vi "主界面.vi"(0 "开始":bool, 5 "打开":bool, 9 "步骤":string[][](table)) -> (4 "T(cool)℃":string, 6 "P（eq)mv":string, 8 "多位阀的位置":string, 10 "R(Gas)mv":string, 15 "F(Flow)ml/min":string)   [LabVIEW 2016]
uses:
  <vilib>/Utility/miscctls.llb/LVRowAndColumnTypeDef.ctl
  <vilib>/Utility/file.llb/Write Delimited Spreadsheet (string).vi
  <vilib>/Utility/file.llb/Read Delimited Spreadsheet (string).vi
panel:
  out "报警":i32=1
  out "蠕动泵":i32=1
  out "电磁阀2":i32=1
  out "电磁阀1":i32=1
  out "气泵":i32=1
  out "时间":string
  out "d15N":string
  out "d15NA":string
  out "N2O":string
  out "d18O":string
  out "H2O  2":string
  out "温度摄氏度":string
  out "d15NB":string
  out "气压Torr":string
  out "超时us":string
  out "航向":string
  out "经度":string
  out "UTC日期":string
  out "速率":string
  out "纬度":string
  out "UTC时间":string
  out "定位信息":string
  in  "数据存储时间间隔（分钟）":dbl format="%#g"
  out "x*y":i32
  in  "数据数组":string[][](array[string])
  in  "停止":bool
  out "Delta2Min":string
  out "H2O":string
  out "12CO2":string
  out "12CO2(dry）":string
  out "13CO2":string
  out "13CO2（dry）":string
  out "Delta5Min":string
  out "Temperature":string
  out "Conductivity":string
  out "Salinity":string
  in  "设备配置&联机":bool
  out "跳转次数变量":i32=2
  out "当前步骤":i32
  in  "添加的数组 2":string[](array[string])
  out "编辑位置":T1
  in  "保存":bool
  in  "插入":bool
  in  "下移":bool
  in  "上移":bool
  in  "删除":bool
  out "数值 2":i32
  out "活动单元格:活动单元格":T1 caption="行和列"
  out "输出数组 2":string[][](array[string])
  in  "簇":T2
  in  "增加":bool
  in  "停止":bool
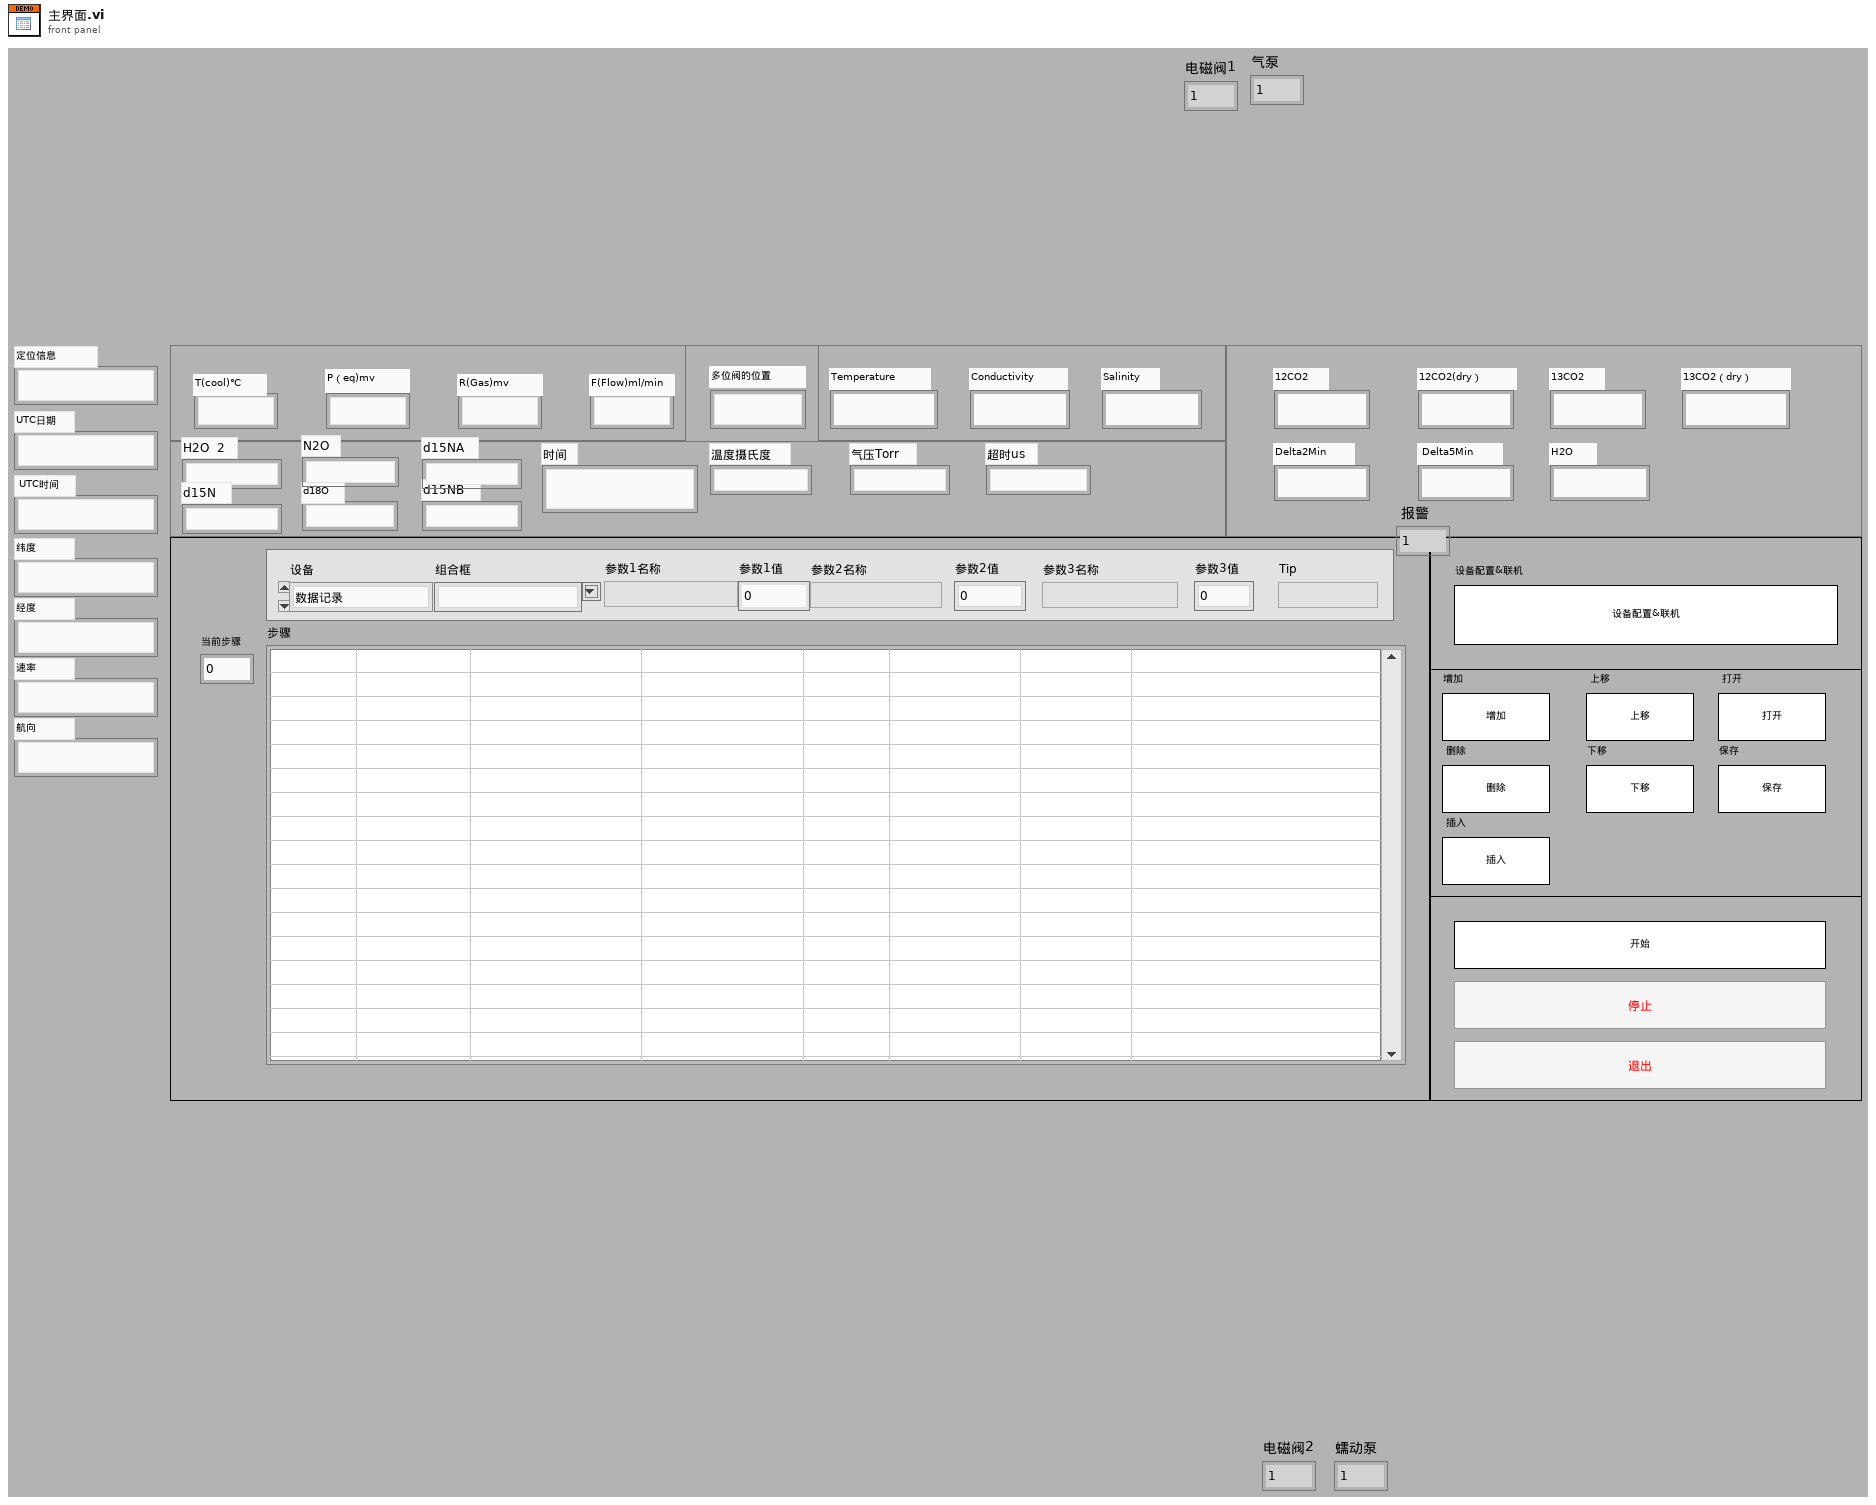
[diagram p1: front panel]
types:
  T1 = typedef "LVRowAndColumnTypeDef.ctl" = cluster{"Row":i32, "Column":i32}
  T2 = cluster{"设备":enum16{"数据记录", "Module", "VICI Valve", "其他"}, "组合框":string, "参数1名称":string, "参数1值":dbl, "参数2名称":string, "参数2值 ":dbl, "参数3名称 ":string, "参数3值  ":dbl, "Tip":string}
  T3 = typedef "LVPoint32TypeDef.ctl" = cluster{"Horizontal":i32, "Vertical":i32}
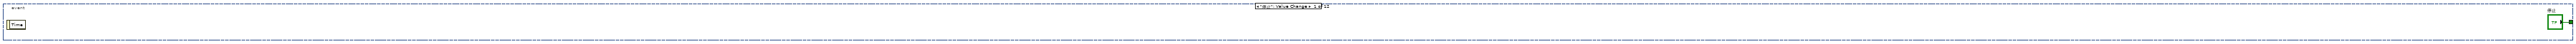
[diagram p2: hidden frame]
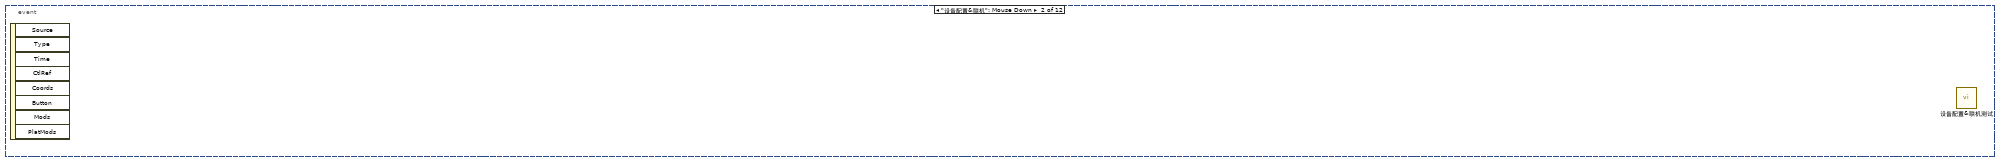
[diagram p3: hidden frame]
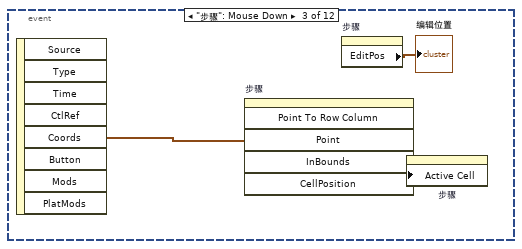
[diagram p4: hidden frame]
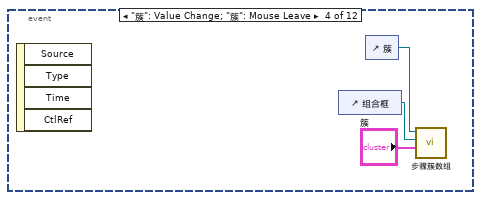
[diagram p5: hidden frame]
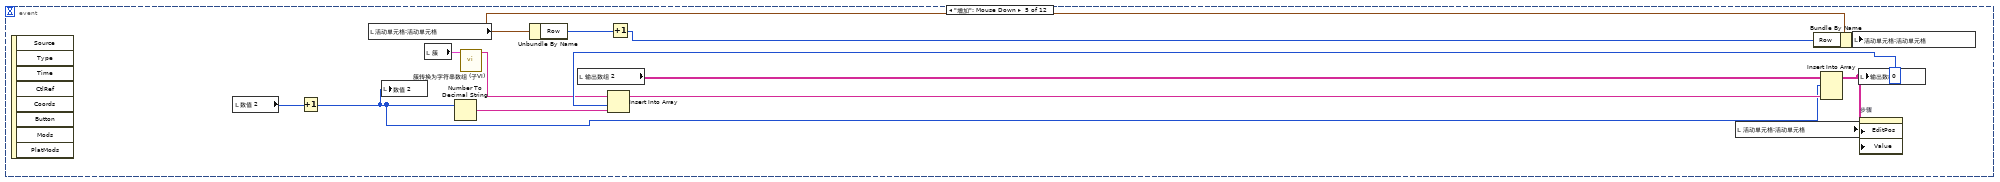
[diagram p6: hidden frame]
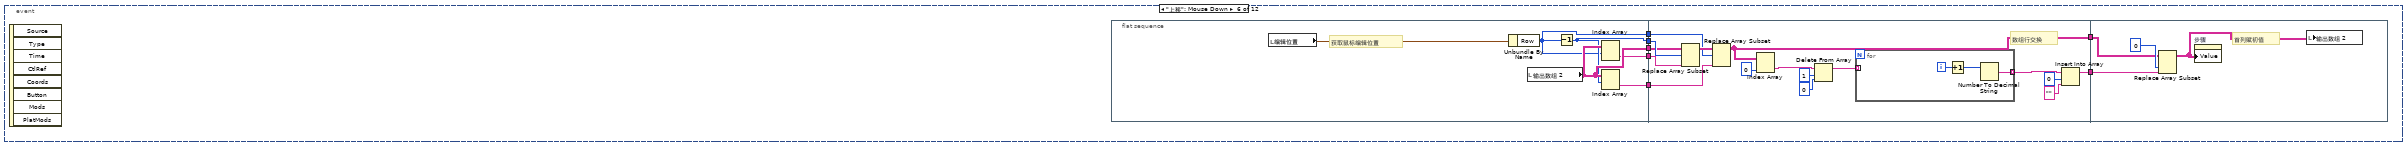
[diagram p7: hidden frame]
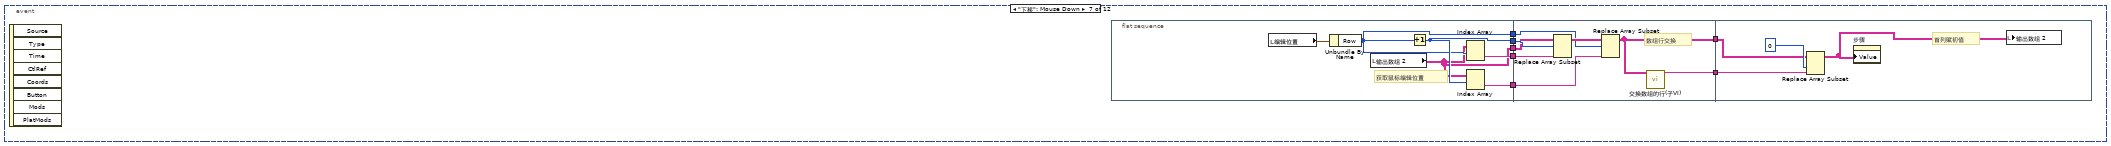
[diagram p8: hidden frame]
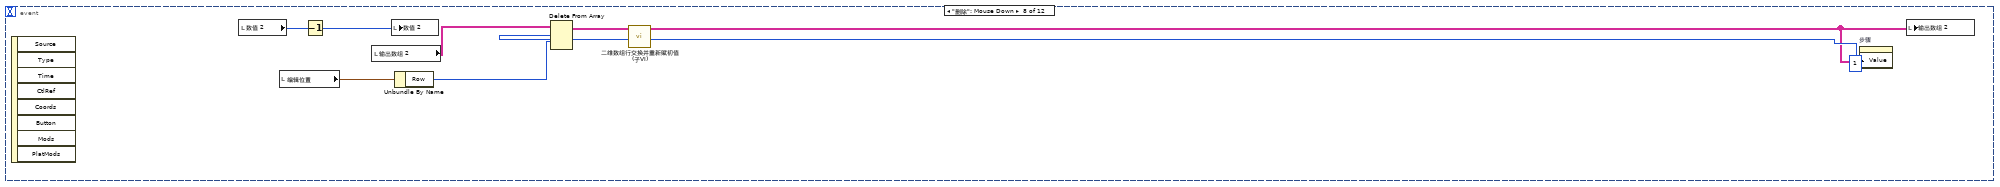
[diagram p9: hidden frame]
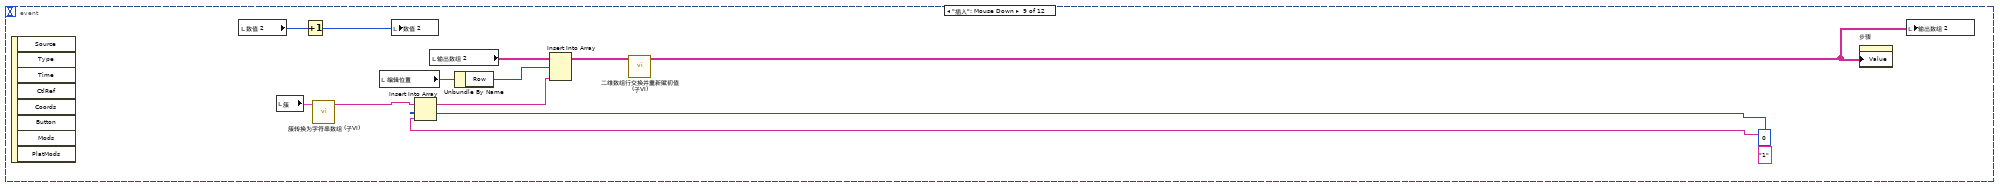
[diagram p10: hidden frame]
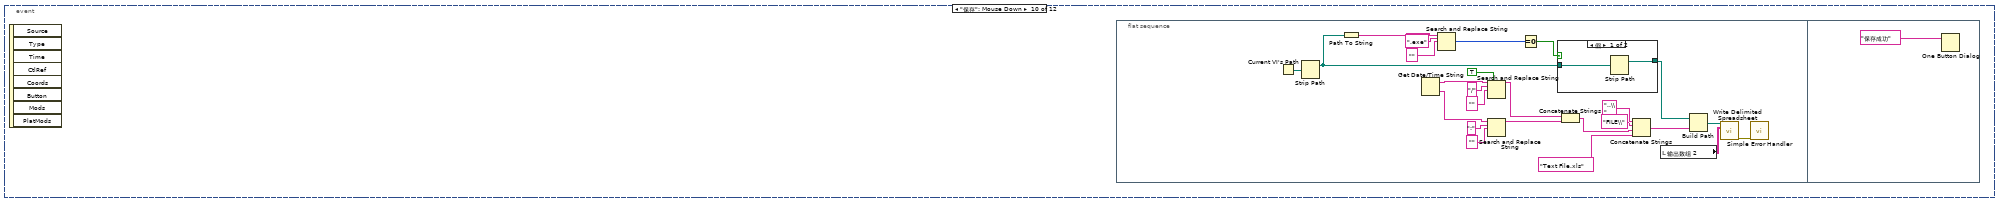
[diagram p11: hidden frame]
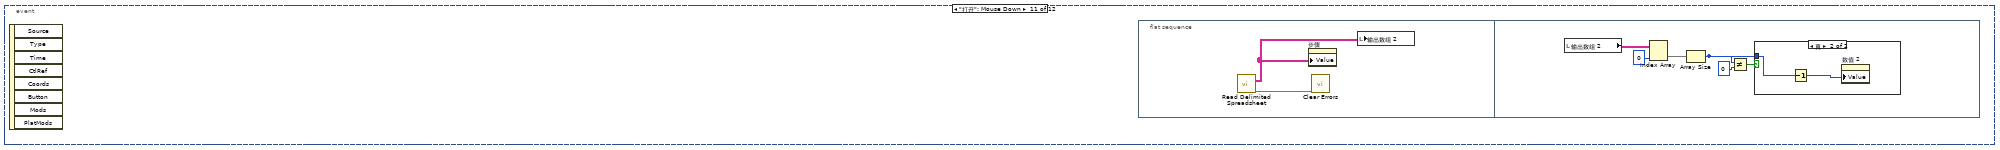
[diagram p13: hidden frame]
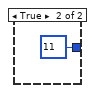
[diagram p15: hidden frame]
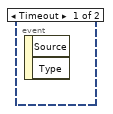
[diagram p17: hidden frame]
diagram:
  # "数组初始化"
  n1 = while {
    stop <- w40 stop-if-true
    w6 = FALSE ("停止")
    n2 = Wait (ms)(milliseconds to wait=u32 300 ("等待时间（毫秒）")) -> ()  [unwired: 1 out]
    n3 = event shown="[11] \"开始\": 鼠标按下" {
      selector: _ -> [_ _ _ _ _ _ _ _ _ _ _ _]
      dyn-events: _ -> [_ _ _ _ _ _ _ _ _ _ _ _]
      timeout: _ -> [_ _ _ _ _ _ _ _ _ _ _ _]
      tunnel: ["停止" _ _ _ _ _ _ _ _ _ _ _] -> w40
      event "停止": Value Change {
        n4 = event-data() -> ()  [unwired: 1 in, 1 out]
      }
      event "设备配置&联机": Mouse Down {
        n5 = event-data() -> ()  [unwired: 1 in, 8 out]
        n6 = call "设备配置&联机测试.vi"() -> ()  [unwired: 11 in, 1 out]
      }
      event "步骤": Mouse Down {
        n7 = event-data() -> ("Coords"=w44:T3)  [unwired: 1 in, 7 out]
        n8 = invoke on="步骤" class="Tbl (严格)" method="Point To Row Column"("Point"=w44) -> ("CellPosition"=w43:T1)  [unwired: 5 in, 5 out]
        n9 = property on="步骤" class="Tbl (严格)"() -> ("EditPos"=→"编辑位置":T1)  [unwired: 2 in, 2 out]
        n10 = property on="步骤" class="Tbl (严格)"("Active Cell"=w43) -> ()  [unwired: 2 in, 2 out]
      }
      event "簇": Value Change; "簇": Mouse Leave {
        n11 = event-data() -> ()  [unwired: 1 in, 4 out]
        n12 = control-ref of="组合框"() -> (w45:refnum<vi>)
        n13 = control-ref of="簇"() -> (w46:refnum<vi>)
        n14 = call "步骤簇数组.vi"("簇"="簇", "组合框"=w45, "簇 2"=w46) -> ()  [unwired: 9 in]
      }
      event "增加": Mouse Down {
        n15 = event-data() -> ()  [unwired: 1 in, 8 out]
        n16 = local read "数值 2"() -> (w53:i32)
        n17 = Increment(x=w53) -> (x+1=w52:i32)
        n18 = local read "活动单元格:活动单元格"() -> (w57:T1)
        n19 = local write "数值 2"(w52) -> ()
        n20 = local read "簇"() -> (w61:T2)
        n21 = Number To Decimal String(number=w52) -> (decimal integer string=w55:string)  [unwired: 1 in]
        n22 = call "簇转换为字符串数组 (子VI).vi"("簇"=w61) -> ("数组"=w48:string[])  [unwired: 10 in]
        n23 = Unbundle By Name(w57) -> ("Row"=w59:i32)
        n24 = local read "输出数组 2"() -> (w49:string[][])
        n25 = Insert Into Array(array=w48, index=0 ("索引"), new element=w55) -> (w54:string[])
        n26 = Increment(x=w59) -> (x+1=w56:i32)
        n27 = local read "活动单元格:活动单元格"() -> (w60:T1)
        n28 = Bundle By Name(cluster=w57, "Row"=w56) -> (w58:T1)
        n29 = Insert Into Array(array=w49, index (row)=w52, new element=w54) -> (w51:string[][])  [unwired: 1 in]
        n30 = local write "活动单元格:活动单元格"(w58) -> ()
        n31 = local write "输出数组 2"(w51) -> ()
        n32 = property on="步骤" class="Tbl (严格)"("EditPos"=w60, "Value"=w51) -> ()  [unwired: 2 in, 2 out]
      }
      event "上移": Mouse Down {
        n33 = event-data() -> ()  [unwired: 1 in, 8 out]
        n34 = flat-sequence {
          tunnel: [w73] -> w68
          tunnel: [w72] -> w67
          tunnel: [w71] -> w66
          tunnel: [w70] -> w65
          tunnel: [w69] -> w64
          tunnel: w68 -> [w77]
          tunnel: w67 -> [w90]
          tunnel: w66 -> [w89]
          tunnel: w65 -> [w87]
          tunnel: w64 -> [w86]
          tunnel: [w75] -> w63
          tunnel: [w76] -> w62
          tunnel: w63 -> [w96]
          tunnel: w62 -> [w95]
          frame #0 {
            # "获取鼠标编辑位置"
            n35 = local read "编辑位置"() -> (w74:T1)
            n36 = Unbundle By Name(w74) -> ("Row"=w69:i32)
            n37 = local read "输出数组 2"() -> (w73:string[][])
            n38 = Decrement(x=w69) -> (x-1=w71:i32)
            n39 = Index Array(array=w73, index (row)=w69) -> (element=w72:string[])  [unwired: 1 in]
            n40 = Index Array(array=w73, index (row)=w71) -> (element=w70:string[])  [unwired: 1 in]
          }
          frame #1 {
            # "数组行交换"
            n41 = Replace Array Subset(array=w77, new element=w90, index (row)=w89) -> (w88:string[][])  [unwired: 1 in]
            n42 = Replace Array Subset(array=w88, new element=w87, index (row)=w86) -> (w75:string[][])  [unwired: 1 in]
            n43 = Index Array(array=w75, index (col)=0 ("禁用的索引 (列)")) -> (element=w84:string[])  [unwired: 1 in]
            n44 = Delete From Array(array=w84, length=1 ("长度"), index=0 ("索引")) -> (array with subset deleted=w81:string[])  [unwired: 1 out]
            n45 = for {
              tunnel: w81 -> [_] mode=indexing
              tunnel: [w91] -> w80 mode=indexing
              i -> [w93]
              n46 = Increment(x=w93) -> (x+1=w92:i32)
              n47 = Number To Decimal String(number=w92) -> (decimal integer string=w91:string)  [unwired: 1 in]
            }
            n48 = Insert Into Array(array=w80, index=0 ("索引"), new element="" ("新元素/子数组")) -> (w76:string[])
          }
          frame #2 {
            # "首列赋初值"
            n49 = Replace Array Subset(array=w96, new element=w95, index (col)=0 ("禁用的索引 (列)")) -> (w94:string[][])  [unwired: 1 in]
            n50 = property on="步骤" class="Tbl (严格)"("Value"=w94) -> ()  [unwired: 2 in, 2 out]
            n51 = local write "输出数组 2"(w94) -> ()
          }
        }
      }
      event "下移": Mouse Down {
        n52 = event-data() -> ()  [unwired: 1 in, 8 out]
        n53 = flat-sequence {
          tunnel: [w105] -> w104
          tunnel: [w110] -> w103
          tunnel: [w109] -> w102
          tunnel: [w108] -> w101
          tunnel: [w107] -> w100
          tunnel: w104 -> [w113]
          tunnel: w103 -> [w118]
          tunnel: w102 -> [w117]
          tunnel: w101 -> [w115]
          tunnel: w100 -> [w114]
          tunnel: [w111] -> w99
          tunnel: [w112] -> w98
          tunnel: w99 -> [w121]
          tunnel: w98 -> [w120]
          frame #0 {
            # "获取鼠标编辑位置"
            n54 = local read "编辑位置"() -> (w106:T1)
            n55 = Unbundle By Name(w106) -> ("Row"=w107:i32)
            n56 = local read "输出数组 2"() -> (w105:string[][])
            n57 = Increment(x=w107) -> (x+1=w109:i32)
            n58 = Index Array(array=w105, index (row)=w107) -> (element=w110:string[])  [unwired: 1 in]
            n59 = Index Array(array=w105, index (row)=w109) -> (element=w108:string[])  [unwired: 1 in]
          }
          frame #1 {
            # "数组行交换"
            n60 = Replace Array Subset(array=w113, new element=w118, index (row)=w117) -> (w116:string[][])  [unwired: 1 in]
            n61 = Replace Array Subset(array=w116, new element=w115, index (row)=w114) -> (w111:string[][])  [unwired: 1 in]
            n62 = call "交换数组的行(子VI).vi"("输出数组输入"=w111) -> ("数组"=w112:string[])  [unwired: 10 in]
          }
          frame #2 {
            # "首列赋初值"
            n63 = Replace Array Subset(array=w121, new element=w120, index (col)=0 ("禁用的索引 (列)")) -> (w119:string[][])  [unwired: 1 in]
            n64 = property on="步骤" class="Tbl (严格)"("Value"=w119) -> ()  [unwired: 2 in, 2 out]
            n65 = local write "输出数组 2"(w119) -> ()
          }
        }
      }
      event "删除": Mouse Down {
        n66 = event-data() -> ()  [unwired: 1 in, 8 out]
        n67 = local read "数值 2"() -> (w126:i32)
        n68 = local read "编辑位置"() -> (w130:T1)
        n69 = Decrement(x=w126) -> (x-1=w125:i32)
        n70 = local read "输出数组 2"() -> (w129:string[][])
        n71 = local write "数值 2"(w125) -> ()
        n72 = Unbundle By Name(w130) -> ("Row"=w127:i32)
        n73 = Delete From Array(array=w129, length=1 ("长度"), index (row)=w127) -> (array with subset deleted=w124:string[][])  [unwired: 1 in, 1 out]
        n74 = call "二维数组行交换并重新赋初值 (子VI).vi"("输出数组 3"=w124) -> ("输出数组 2"=w123:string[][])  [unwired: 10 in]
        n75 = property on="步骤" class="Tbl (严格)"("Value"=w123) -> ()  [unwired: 2 in, 2 out]
        n76 = local write "输出数组 2"(w123) -> ()
      }
      event "插入": Mouse Down {
        n77 = event-data() -> ()  [unwired: 1 in, 8 out]
        n78 = local read "数值 2"() -> (w132:i32)
        n79 = local read "簇"() -> (w137:T2)
        n80 = Increment(x=w132) -> (x+1=w131:i32)
        n81 = call "簇转换为字符串数组 (子VI).vi"("簇"=w137) -> ("数组"=w136:string[])  [unwired: 10 in]
        n82 = local read "编辑位置"() -> (w142:T1)
        n83 = local write "数值 2"(w131) -> ()
        n84 = Insert Into Array(array=w136, index=0 ("索引"), new element="1" ("新元素/子数组")) -> (w133:string[])
        n85 = local read "输出数组 2"() -> (w141:string[][])
        n86 = Unbundle By Name(w142) -> ("Row"=w140:i32)
        n87 = Insert Into Array(array=w141, index (row)=w140, new element=w133) -> (w139:string[][])  [unwired: 1 in]
        n88 = call "二维数组行交换并重新赋初值 (子VI).vi"("输出数组 3"=w139) -> ("输出数组 2"=w138:string[][])  [unwired: 10 in]
        n89 = property on="步骤" class="Tbl (严格)"("Value"=w138) -> ()  [unwired: 2 in, 2 out]
        n90 = local write "输出数组 2"(w138) -> ()
      }
      event "保存": Mouse Down {
        n91 = event-data() -> ()  [unwired: 1 in, 8 out]
        n92 = flat-sequence {
          frame #0 {
            n93 = Current VI's Path() -> (path=w152:path)
            n94 = Strip Path(path=w152) -> (stripped path=w144:path)  [unwired: 1 out]
            n95 = Path To String(path=w144) -> (string=w149:string)
            n96 = Get Date/Time String() -> (date string=w160:string, time string=w163:string)  [unwired: 3 in]
            n97 = Search and Replace String(input string=w149, search string=".exe" ("搜索字符串"), replace string="" ("替换字符串(\"\")")) -> (number of replacements=w146:i32)  [unwired: 5 in, 3 out]
            n98 = Search and Replace String(input string=w163, search string=":" ("搜索字符串"), replace string="" ("替换字符串(\"\")")) -> (result string=w155:string)  [unwired: 5 in, 3 out]
            n99 = Search and Replace String(replace all?=TRUE ("替换全部？(F)"), input string=w160, search string="/" ("搜索字符串"), replace string="" ("替换字符串(\"\")")) -> (result string=w156:string)  [unwired: 4 in, 3 out]
            n100 = Equal To 0?(x=w146) -> (x = 0?=w145:bool)
            n101 = case shown="假" w145 {
              tunnel: w144 -> [w169 w170]
              tunnel: [w168 w170] -> w143
              frame False {
                n102 = Strip Path(path=w169) -> (stripped path=w168:path)  [unwired: 1 out]
              }
              frame True {
              }
            }
            n103 = Concatenate Strings(w156, w155) -> (w154:string)
            n104 = Concatenate Strings("..\\" ("字符串"), "FILE\\" ("替换字符串(\"\")"), w154, "Text File.xls" ("name or relative path")) -> (w165:string)
            n105 = local read "输出数组 2"() -> (w167:string[][])
            n106 = Build Path(base path=w143, name or relative path=w165) -> (appended path=w166:path)
            n107 = call-poly <vilib>:"Write Delimited Spreadsheet.vi"("file path (dialog if empty)"=w166, "2D data"=w167) -> ("error out"=w153:errorcluster)  [unwired: 12 in, 1 out]
            n108 = call <vilib>:"Simple Error Handler.vi"("error in (no error)"=w153) -> ()  [unwired: 4 in, 5 out]
          }
          frame #1 {
            n109 = One Button Dialog(message="保存成功" ("消息")) -> ()  [unwired: 1 in, 1 out]
          }
        }
      }
      event "打开": Mouse Down {
        n110 = event-data() -> ()  [unwired: 1 in, 8 out]
        n111 = flat-sequence {
          frame #0 {
            n112 = call-poly <vilib>:"Read Delimited Spreadsheet.vi"() -> ("all rows"=w173:string[][], "error out"=w172:errorcluster)  [unwired: 10 in, 4 out]
            n113 = property on="步骤" class="Tbl (严格)"("Value"=w173) -> ()  [unwired: 2 in, 2 out]
            n114 = call <vilib>:"Clear Errors.vi"("error in (no error)"=w172) -> ()  [unwired: 5 in, 2 out]
            n115 = local write "输出数组 2"(w173) -> ()
          }
          frame #1 {
            n116 = local read "输出数组 2"() -> (w177:string[][])
            n117 = Index Array(array=w177, index (col)=0 ("禁用的索引 (列)")) -> (element=w175:string[])  [unwired: 1 in]
            n118 = Array Size(array=w175) -> (size(s)=w174:i32)
            n119 = Not Equal?(x=w174, y=u32 0) -> (x != y?=w178:bool)
            n120 = case shown="真" w178 {
              tunnel: w174 -> [_ w181]
              frame False {
              }
              frame True {
                n121 = Decrement(x=w181) -> (x-1=w180:i32)
                n122 = property on="数值 2" class="DigNum (严格)"("Value"=w180) -> ()  [unwired: 2 in, 2 out]
              }
            }
          }
        }
      }
      event "开始": Mouse Down {
        w182 = 0 ("气泵")
        w184 = ""
        n123 = event-data() -> ()  [unwired: 1 in, 8 out]
        n124 = while {
          stop <- w215 stop-if-true
          # "数据显示"
          # "读取流量传感器"
          n125 = call "读取流量传感器(子VI).vi"() -> ("结果"=w216:bool, "R(Gas)mv"=w221:string, "F(Flow)ml/min"=w220:string, "P（eq)mv"=w222:string, "T(cool)℃"=w223:string)  [unwired: 7 in]
          n126 = local write "P（eq)mv"(w222) -> ()
          n127 = local write "R(Gas)mv"(w221) -> ()
          n128 = local write "F(Flow)ml/min"(w220) -> ()
          n129 = local write "T(cool)℃"(w223) -> ()
          n130 = disable-structure shown="禁用" {
            frame Disabled {
              n131 = call "N2O同位素分析仪串口通讯.vi"("VISA resource name"=refnum<visa-resource-name> "COM8") -> ("温度摄氏度"=→"温度摄氏度":string, "d15NB"=→"d15NB":string, "时间"=→"时间":string, "N2O"=→"N2O":string, "d15N"=→"d15N":string, "d18O"=→"d18O":string, "超时us"=→"超时us":string, "气压Torr"=→"气压Torr":string, "H2O"=→"H2O  2":string, "d15NA"=→"d15NA":string)  [unwired: 5 in]
            }
            frame Enabled {
            }
          }
          n132 = call "SBE45通讯参数 (子VI).vi"() -> ("错误输出"=w214:errorcluster, "Salinity"=w238:string, "Conductivity"=w239:string, "Temperature"=w240:string)  [unwired: 8 in]
          "Temperature" <- w240
          "Conductivity" <- w239
          "Salinity" <- w238
          n133 = call "G2131-i通讯参数 (子VI).vi"() -> ("12CO2(dry）"=w235:string, "Delta2Min"=w231:string, "12CO2"=w236:string, "Delta5Min"=w230:string, "H2O"=w232:string, "13CO2"=w234:string, "13CO2（dry）"=w233:string)  [unwired: 5 in]
          "Delta2Min" <- w231
          "H2O" <- w232
          "12CO2" <- w236
          "12CO2(dry）" <- w235
          "13CO2" <- w234
          "13CO2（dry）" <- w233
          "Delta5Min" <- w230
          n134 = local read "多位阀的位置"() -> (w241:string)
          n135 = Get Date/Time String(want seconds? (F)=TRUE ("需要秒？(F)")) -> (date string=w227:string, time string=w229:string)  [unwired: 2 in]
          n136 = Concatenate Strings(w227, " " ("字符串"), w229) -> (w205:string)
          n137 = call "GPS-1仪器串口通讯.vi"("VISA resource name"=refnum<visa-resource-name> "COM5", "baud rate (9600)"=u32 9600) -> ("速率"=w211:string, "经度"=w210:string, "定位信息"=w206:string, "UTC日期"=w207:string, "航向"=w212:string, "UTC时间"=w208:string, "纬度"=w209:string)  [unwired: 10 in, 1 out]
          "定位信息" <- w206
          "UTC时间" <- w208
          "纬度" <- w209
          "速率" <- w211
          "UTC日期" <- w207
          "经度" <- w210
          "航向" <- w212
          n138 = Compound Arithmetic op=OR ("复合运算")(w214, w216, "停止") -> (w215:bool)
          n139 = Build Array(w205, w206, w207, w208, w209, w210, w211, w212, w223, w222, w221, w220, w241, w240, w239, w238, w236, w235, w234, w233, w232, w231, w230) -> (w237:string[])
          n140 = Insert Into Array(array="数据数组", index (row)=2 ("索引 (行)"), new element=w237) -> (w213:string[][])  [unwired: 1 in]
          n141 = local write "数据数组"(w213) -> ()
          n142 = case shown="假" "停止" {
            tunnel: [w242 11 ("x*y")] -> w217
            frame False {
              n143 = local read "x*y"() -> (w242:i32)
            }
            frame True {
            }
          }
          n144 = Wait (ms)(milliseconds to wait=w217) -> ()  [unwired: 1 out]
        }
        n145 = local read "输出数组 2"() -> (w203:string[][])
        n146 = local write "F(Flow)ml/min"(w184) -> ()
        n147 = local write "P（eq)mv"(w184) -> ()
        n148 = local write "T(cool)℃"(w184) -> ()
        n149 = local write "R(Gas)mv"(w184) -> ()
        n150 = call "提示用户输入"() -> ("数据存储时间间隔（分钟）"=w183:dbl)  [unwired: 17 in, 2 out]
        n151 = call "二维数组行交换并重新赋初值 (子VI).vi"("输出数组 3"=w203) -> ("输出数组 2"=w202:string[][])  [unwired: 10 in]
        n152 = Delete From Array(array=w202, index (row)=0 ("索引 (行)")) -> (array with subset deleted=w190:string[][])  [unwired: 2 in, 1 out]
        n153 = local write "数据存储时间间隔（分钟）"(w183) -> ()
        n154 = Index Array(array=w190, index (col)=2 ("禁用的索引 (列)")) -> (element=w199:string[])  [unwired: 1 in]
        n155 = Index Array(array=w190, index (col)=4 ("禁用的索引 (列)")) -> (element=w200:string[])  [unwired: 1 in]
        n156 = Index Array(array=w190, index (col)=6 ("禁用的索引 (列)")) -> (element=w188:string[])  [unwired: 1 in]
        n157 = local write "电磁阀2"(w182) -> ()
        n158 = local write "电磁阀1"(w182) -> ()
        n159 = local write "报警"(w182) -> ()
        n160 = local write "蠕动泵"(w182) -> ()
        n161 = local write "气泵"(w182) -> ()
        n162 = Build Array(w199, w200, w188) -> (w192:string[][])
        n163 = Obtain Queue(name (unnamed)="步骤执行顺序数组" ("名称（未命名）"), element data type="添加的数组 2") -> (queue out=w193:refnum<queue>, error out=w186:errorcluster)  [unwired: 3 in, 1 out]
        n164 = while {
          tunnel: w192 -> [w325]
          tunnel: [w323] -> w194
          tunnel: w193 -> [w318]
          tunnel: w186 -> [w296]
          tunnel: [w287] -> w185
          stop <- w255 stop-if-true
          n165 = event shown="[1] \"当前步骤\": 值改变" {
            selector: _ -> [_ _]
            dyn-events: _ -> [_ _]
            timeout: _ -> [_ _]
            event Timeout {
              n166 = event-data() -> ()  [unwired: 1 in, 2 out]
            }
            event "当前步骤": Value Change {
              n167 = event-data() -> ()  [unwired: 1 in, 6 out]
              n168 = control-ref of="步骤"() -> (w328:refnum<vi>)
              n169 = property on="当前步骤" class="DigNum (严格)"() -> ("Value"=w327:i32)  [unwired: 2 in, 2 out]
              n170 = Bundle By Name(cluster=T1 {"Row"=0, "Column"=-2} ("活动单元格:活动单元格"), "Row"=w327) -> (w331:T1)
              n171 = property class="Tbl (严格)"(reference=w328, "Cell BG Color"=u32 16448250, "Active Cell"=w331, "Cell BG Color"=u32 3381759) -> ()  [unwired: 1 in, 2 out]
            }
          }
          n172 = Get Queue Status(queue=w318) -> ()  [unwired: 2 in, 8 out]
          n173 = Wait (ms)(milliseconds to wait=u32 3000 ("等待时间（毫秒）")) -> ()  [unwired: 1 out]
          n174 = local read "当前步骤"() -> (w319:i32)
          n175 = Index Array(array=w325, index (col)=w319) -> (element=w317:string[])  [unwired: 1 in]
          n176 = Increment(x=w319) -> (x+1=w258:i32)
          n177 = Empty Array?(array=w317) -> (empty?=w259:bool)
          n178 = Enqueue Element(queue=w318, element=w317, error in (no error)=w296) -> (queue out=w326:refnum<queue>, error out=w297:errorcluster)  [unwired: 1 in, 1 out]
          n179 = property on="当前步骤" class="DigNum (严格)"("Val(Sgnl)"=w258) -> ()  [unwired: 2 in, 2 out]
          n180 = Dequeue Element(queue=w326, error in (no error)=w297) -> (queue out=w323:refnum<queue>, element=w265:string[], error out=w287:errorcluster)  [unwired: 1 in, 1 out]
          n181 = Index Array(array=w265, index=0 ("索引")) -> (element=w262:string)
          n182 = Equal?(x=w262, y="Control Devices") -> (x = y?=w274:bool)
          n183 = Equal?(x=w262, y="Read Alarm ") -> (x = y?=w270:bool)
          n184 = Equal?(x=w262, y="Set Valve Position") -> (x = y?=w303:bool)
          n185 = Equal?(x=w262, y="Read All sensor Values") -> (x = y?=w304:bool)
          n186 = Equal?(x=w262, y="暂停") -> (x = y?=w261:bool)
          n187 = Equal?(x=w262, y="恢复") -> (x = y?=w260:bool)
          n188 = Equal?(x=w262, y="等待") -> (x = y?=w299:bool)
          n189 = Equal?(x=w262, y="开始") -> (x = y?=w266:bool)
          n190 = Equal?(x=w262, y="跳转事件") -> (x = y?=w320:bool)
          n191 = Equal?(x=w262, y="气泵1、2") -> (x = y?=w316:bool)
          n192 = Equal?(x=w262, y="电磁阀1") -> (x = y?=w315:bool)
          n193 = Equal?(x=w262, y="电磁阀2") -> (x = y?=w312:bool)
          n194 = Equal?(x=w262, y="蠕动泵") -> (x = y?=w311:bool)
          n195 = Equal?(x=w262, y="报警器开") -> (x = y?=w308:bool)
          n196 = Equal?(x=w262, y="报警器关") -> (x = y?=w307:bool)
          n197 = Equal?(x=w262, y="单次记录") -> (x = y?=w268:bool)
          n198 = Or(x=w274, y=w270) -> (x .or. y?=w273:bool)
          n199 = case shown="真" w311 {
            tunnel: w265 -> [_ w478]
            tunnel: [_ w476] -> w293
            frame False {
            }
            frame True {
              # "蠕动泵"
              n200 = Index Array(array=w478, index=1 ("索引")) -> (element=w480:string)
              n201 = Equal?(x=w480, y="1") -> (x = y?=w477:bool)
              n202 = case shown="真" w477 {
                tunnel: [_ w497] -> w476
                tunnel: [0 ("电磁阀1") 10 ("电磁阀1")] -> w475
                frame False {
                  n203 = disable-structure shown="禁用" {
                    disable-tunnel: [w483 _] -> _
                    frame Disabled {
                      n204 = call "Module仪器串口通讯.vi"("输入指令"="$3DO00\r", "baud rate"=u32 300 ("baud rate (9600)"), "VISA resource name"=refnum<visa-resource-name> "COM3") -> ("错误输出"=w483:errorcluster)  [unwired: 2 out]
                    }
                    frame Enabled {
                    }
                  }
                }
                frame True {
                  n205 = control-ref of="电磁阀2"() -> (w493:refnum<vi>)
                  n206 = control-ref of="电磁阀1"() -> (w495:refnum<vi>)
                  n207 = control-ref of="报警"() -> (w494:refnum<vi>)
                  n208 = control-ref of="气泵"() -> (w492:refnum<vi>)
                  n209 = call "数值连接 (子VI).vi"("DigNum引用句柄 4"=w495, "x"=10, "DigNum引用句柄 3"=w494, "DigNum引用句柄输入"=w493, "Digital输入"=w492) -> ("数据字符串"=w490:string)  [unwired: 6 in]
                  n210 = Replace Substring(2:2 ("长度（子字符串长度）"), 3:4 ("偏移量(0)"), 4:w490, 5:"$3DO10\r" ("输入指令")) -> (1:w489:string)  [unwired: 1 out]
                  n211 = call "Module仪器串口通讯.vi"("输入指令"=w489, "baud rate"=u32 300 ("baud rate (9600)"), "VISA resource name"=refnum<visa-resource-name> "COM3") -> ("错误输出"=w497:errorcluster)  [unwired: 2 out]
                }
              }
              "蠕动泵" <- w475
            }
          }
          n212 = case shown="真" w261 {
            frame False {
            }
            frame True {
              n213 = local read "当前步骤"() -> (w336:i32)
              n214 = Increment(x=w336) -> (x+1=w335:i32)
              n215 = property on="当前步骤" class="DigNum (严格)"("Val(Sgnl)"=w335) -> ()  [unwired: 2 in, 2 out]
            }
          }
          n216 = case shown="真" w260 {
            frame False {
            }
            frame True {
              n217 = local read "当前步骤"() -> (w334:i32)
              n218 = Increment(x=w334) -> (x+1=w333:i32)
              n219 = property on="当前步骤" class="DigNum (严格)"("Val(Sgnl)"=w333) -> ()  [unwired: 2 in, 2 out]
            }
          }
          n220 = case shown="真" w273 {
            frame False {
            }
            frame True {
              n221 = local read "当前步骤"() -> (w387:i32)
              n222 = Increment(x=w387) -> (x+1=w386:i32)
              n223 = property on="当前步骤" class="DigNum (严格)"("Val(Sgnl)"=w386) -> ()  [unwired: 2 in, 2 out]
            }
          }
          n224 = case shown="真" w299 {
            tunnel: w265 -> [_ w392]
            frame False {
            }
            frame True {
              n225 = Index Array(array=w392, index=1 ("索引")) -> (element=w391:string)
              n226 = Decimal String To Number(string=w391) -> (number=w390:i32)  [unwired: 2 in, 1 out]
              n227 = Multiply(x=w390, y=60000) -> (x*y=w388:i32)
              n228 = Wait (ms)(milliseconds to wait=w388) -> ()  [unwired: 1 out]
            }
          }
          n229 = case shown="真" w316 {
            tunnel: w265 -> [_ w554]
            tunnel: [_ w552] -> w298
            frame False {
            }
            frame True {
              # "气泵"
              n230 = Index Array(array=w554, index=1 ("索引")) -> (element=w556:string)
              n231 = Equal?(x=w556, y="1") -> (x = y?=w553:bool)
              n232 = case shown="真" w553 {
                tunnel: [_ w574] -> w552
                tunnel: [0 1] -> w551
                frame False {
                  n233 = disable-structure shown="禁用" {
                    disable-tunnel: [w559 _] -> _
                    frame Disabled {
                      n234 = call "Module仪器串口通讯.vi"("输入指令"="$3DO00\r", "baud rate"=u32 300 ("baud rate (9600)"), "VISA resource name"=refnum<visa-resource-name> "COM3") -> ("错误输出"=w559:errorcluster)  [unwired: 2 out]
                    }
                    frame Enabled {
                    }
                  }
                }
                frame True {
                  n235 = control-ref of="电磁阀2"() -> (w568:refnum<vi>)
                  n236 = control-ref of="电磁阀1"() -> (w569:refnum<vi>)
                  n237 = control-ref of="蠕动泵"() -> (w570:refnum<vi>)
                  n238 = control-ref of="报警"() -> (w571:refnum<vi>)
                  n239 = call "数值连接 (子VI).vi"("DigNum引用句柄 4"=w571, "x"=1, "DigNum引用句柄 3"=w570, "DigNum引用句柄输入"=w569, "Digital输入"=w568) -> ("数据字符串"=w567:string)  [unwired: 6 in]
                  n240 = Replace Substring(2:2 ("长度（子字符串长度）"), 3:4 ("偏移量(0)"), 4:w567, 5:"$3DO01\r" ("输入指令")) -> (1:w564:string)  [unwired: 1 out]
                  n241 = call "Module仪器串口通讯.vi"("输入指令"=w564, "baud rate"=u32 300 ("baud rate (9600)"), "VISA resource name"=refnum<visa-resource-name> "COM3") -> ("错误输出"=w574:errorcluster)  [unwired: 2 out]
                }
              }
              "气泵" <- w551
            }
          }
          n242 = case shown="真" w315 {
            tunnel: w265 -> [_ w529]
            tunnel: [_ w527] -> w291
            frame False {
            }
            frame True {
              # "电磁阀1"
              n243 = Index Array(array=w529, index=1 ("索引")) -> (element=w531:string)
              n244 = Equal?(x=w531, y="1") -> (x = y?=w528:bool)
              n245 = case shown="真" w528 {
                tunnel: [_ w547] -> w527
                tunnel: [0 ("电磁阀1") 4 ("电磁阀1")] -> w526
                frame False {
                  n246 = disable-structure shown="禁用" {
                    frame Disabled {
                      n247 = call "Module仪器串口通讯.vi"("输入指令"="$3DO00\r", "baud rate"=u32 300 ("baud rate (9600)"), "VISA resource name"=refnum<visa-resource-name> "COM3") -> ()  [unwired: 3 out]
                    }
                    frame Enabled {
                    }
                  }
                }
                frame True {
                  n248 = control-ref of="电磁阀2"() -> (w540:refnum<vi>)
                  n249 = control-ref of="蠕动泵"() -> (w541:refnum<vi>)
                  n250 = control-ref of="报警"() -> (w539:refnum<vi>)
                  n251 = control-ref of="气泵"() -> (w542:refnum<vi>)
                  n252 = call "数值连接 (子VI).vi"("DigNum引用句柄 4"=w539, "x"=4, "DigNum引用句柄 3"=w540, "DigNum引用句柄输入"=w541, "Digital输入"=w542) -> ("数据字符串"=w545:string)  [unwired: 6 in]
                  n253 = Replace Substring(2:2 ("长度（子字符串长度）"), 3:4 ("偏移量(0)"), 4:w545, 5:"$3DO04\r" ("输入指令")) -> (1:w538:string)  [unwired: 1 out]
                  n254 = call "Module仪器串口通讯.vi"("输入指令"=w538, "baud rate"=u32 300 ("baud rate (9600)"), "VISA resource name"=refnum<visa-resource-name> "COM3") -> ("错误输出"=w547:errorcluster)  [unwired: 2 out]
                }
              }
              "电磁阀1" <- w526
            }
          }
          n255 = case shown="真" w320 {
            tunnel: w265 -> [_ w577]
            frame False {
            }
            frame True {
              # "跳转次数"
              n256 = Index Array(array=w577, index=2 ("索引")) -> (element=w582:string)
              n257 = local read "跳转次数变量"() -> (w581:i32)
              n258 = Decimal String To Number(string=w582) -> (number=w578:i32)  [unwired: 2 in, 1 out]
              n259 = Increment(x=w581) -> (x+1=w580:i32)
              n260 = local write "跳转次数变量"(w580) -> ()
              n261 = Greater Or Equal?(x=w580, y=w578) -> (x >= y?=w579:bool)
              n262 = case shown="真" w579 {
                tunnel: w577 -> [w584 _]
                frame False {
                  # "跳转"
                  n263 = Index Array(array=w584, index=1 ("索引")) -> (element=w586:string)
                  n264 = Decimal String To Number(string=w586) -> (number=w587:i32)  [unwired: 2 in, 1 out]
                  n265 = property on="当前步骤" class="DigNum (严格)"("Val(Sgnl)"=w587) -> ()  [unwired: 2 in, 2 out]
                }
                frame True {
                  n266 = local read "当前步骤"() -> (w589:i32)
                  n267 = Increment(x=w589) -> (x+1=w588:i32)
                  n268 = property on="当前步骤" class="DigNum (严格)"("Val(Sgnl)"=w588) -> ()  [unwired: 2 in, 2 out]
                }
              }
            }
          }
          n269 = case shown="真" w312 {
            tunnel: w265 -> [_ w504]
            tunnel: [_ w502] -> w292
            frame False {
            }
            frame True {
              # "电磁阀2"
              n270 = Index Array(array=w504, index=1 ("索引")) -> (element=w506:string)
              n271 = Equal?(x=w506, y="1") -> (x = y?=w503:bool)
              n272 = case shown="真" w503 {
                tunnel: [_ w523] -> w502
                tunnel: [0 ("电磁阀1") 8 ("电磁阀1")] -> w501
                frame False {
                  n273 = disable-structure shown="禁用" {
                    frame Disabled {
                      n274 = call "Module仪器串口通讯.vi"("输入指令"="$3DO00\r", "baud rate"=u32 300 ("baud rate (9600)"), "VISA resource name"=refnum<visa-resource-name> "COM3") -> ()  [unwired: 3 out]
                    }
                    frame Enabled {
                    }
                  }
                }
                frame True {
                  n275 = control-ref of="报警"() -> (w512:refnum<vi>)
                  n276 = control-ref of="电磁阀1"() -> (w514:refnum<vi>)
                  n277 = control-ref of="蠕动泵"() -> (w513:refnum<vi>)
                  n278 = control-ref of="气泵"() -> (w515:refnum<vi>)
                  n279 = call "数值连接 (子VI).vi"("DigNum引用句柄 4"=w512, "x"=8, "DigNum引用句柄 3"=w513, "DigNum引用句柄输入"=w514, "Digital输入"=w515) -> ("数据字符串"=w516:string)  [unwired: 6 in]
                  n280 = Replace Substring(2:2 ("长度（子字符串长度）"), 3:4 ("偏移量(0)"), 4:w516, 5:"$3DO08\r" ("输入指令")) -> (1:w521:string)  [unwired: 1 out]
                  n281 = call "Module仪器串口通讯.vi"("输入指令"=w521, "baud rate"=u32 300 ("baud rate (9600)"), "VISA resource name"=refnum<visa-resource-name> "COM3") -> ("错误输出"=w523:errorcluster)  [unwired: 2 out]
                }
              }
              "电磁阀2" <- w501
            }
          }
          n282 = case shown="真" w308 {
            tunnel: w265 -> [_ w452]
            tunnel: [_ w450] -> w294
            frame False {
            }
            frame True {
              # "报警器"
              n283 = Index Array(array=w452, index=1 ("索引")) -> (element=w454:string)
              n284 = Equal?(x=w454, y="1") -> (x = y?=w451:bool)
              n285 = case shown="真" w451 {
                tunnel: [_ w471] -> w450
                tunnel: [0 ("电磁阀1") 40 ("电磁阀1")] -> w449
                frame False {
                  n286 = disable-structure shown="禁用" {
                    disable-tunnel: [w457 _] -> _
                    frame Disabled {
                      n287 = call "Module仪器串口通讯.vi"("输入指令"="$3DO00\r", "baud rate"=u32 300 ("baud rate (9600)"), "VISA resource name"=refnum<visa-resource-name> "COM3") -> ("错误输出"=w457:errorcluster)  [unwired: 2 out]
                    }
                    frame Enabled {
                    }
                  }
                }
                frame True {
                  n288 = control-ref of="电磁阀2"() -> (w468:refnum<vi>)
                  n289 = control-ref of="蠕动泵"() -> (w467:refnum<vi>)
                  n290 = control-ref of="电磁阀1"() -> (w466:refnum<vi>)
                  n291 = control-ref of="气泵"() -> (w469:refnum<vi>)
                  n292 = call "数值连接 (子VI).vi"("DigNum引用句柄 4"=w466, "x"=4, "DigNum引用句柄 3"=w467, "DigNum引用句柄输入"=w468, "Digital输入"=w469) -> ("数据字符串"=w463:string)  [unwired: 6 in]
                  n293 = Replace Substring(2:2 ("长度（子字符串长度）"), 3:4 ("偏移量(0)"), 4:w463, 5:"$3DO40\r" ("输入指令")) -> (1:w465:string)  [unwired: 1 out]
                  n294 = call "Module仪器串口通讯.vi"("输入指令"=w465, "baud rate"=u32 300 ("baud rate (9600)"), "VISA resource name"=refnum<visa-resource-name> "COM3") -> ("错误输出"=w471:errorcluster)  [unwired: 2 out]
                }
              }
              "报警" <- w449
            }
          }
          n295 = case shown="真" w307 {
            tunnel: w265 -> [_ w437]
            tunnel: [_ w435] -> w295
            frame False {
            }
            frame True {
              n296 = Index Array(array=w437, index=1 ("索引")) -> (element=w439:string)
              n297 = Equal?(x=w439, y="1") -> (x = y?=w436:bool)
              n298 = case shown="真" w436 {
                tunnel: [_ w445] -> w435
                frame False {
                  n299 = disable-structure shown="禁用" {
                    disable-tunnel: [w441 _] -> _
                    frame Disabled {
                      n300 = call "Module仪器串口通讯.vi"("输入指令"="$3DO00\r", "baud rate"=u32 300 ("baud rate (9600)"), "VISA resource name"=refnum<visa-resource-name> "COM3") -> ("错误输出"=w441:errorcluster)  [unwired: 2 out]
                    }
                    frame Enabled {
                    }
                  }
                }
                frame True {
                  n301 = call "Module仪器串口通讯.vi"("输入指令"="$3DO80\r", "baud rate"=u32 300 ("baud rate (9600)"), "VISA resource name"=refnum<visa-resource-name> "COM3") -> ("错误输出"=w445:errorcluster)  [unwired: 2 out]
                }
              }
            }
          }
          n302 = case shown="真" w268 {
            frame False {
            }
            frame True {
              n303 = Current VI's Path() -> (path=w381:path)
              n304 = Strip Path(path=w381) -> (stripped path=w359:path)  [unwired: 1 out]
              n305 = Path To String(path=w359) -> (string=w364:string)
              n306 = Get Date/Time String() -> (date string=w375:string, time string=w378:string)  [unwired: 3 in]
              n307 = Search and Replace String(input string=w378, search string=":" ("搜索字符串"), replace string="" ("替换字符串(\"\")")) -> (result string=w370:string)  [unwired: 5 in, 3 out]
              n308 = Search and Replace String(replace all?=TRUE ("替换全部？(F)"), input string=w375, search string="/" ("搜索字符串"), replace string="" ("替换字符串(\"\")")) -> (result string=w371:string)  [unwired: 4 in, 3 out]
              n309 = Search and Replace String(input string=w364, search string=".exe" ("搜索字符串"), replace string="" ("替换字符串(\"\")")) -> (number of replacements=w360:i32)  [unwired: 5 in, 3 out]
              n310 = Concatenate Strings(w371, w370) -> (w369:string)
              n311 = Equal To 0?(x=w360) -> (x = 0?=w361:bool)
              n312 = case shown="假" w361 {
                tunnel: w359 -> [w384 w385]
                tunnel: [w383 w385] -> w358
                frame False {
                  n313 = Strip Path(path=w384) -> (stripped path=w383:path)  [unwired: 1 out]
                }
                frame True {
                }
              }
              n314 = Concatenate Strings("..\\" ("字符串"), "DATA\\" ("字符串"), w369, "Data File.xls" ("name or relative path")) -> (w380:string)
              n315 = local read "数据数组"() -> (w382:string[][])
              n316 = Build Path(base path=w358, name or relative path=w380) -> (appended path=w368:path)
              n317 = call-poly <vilib>:"Write Delimited Spreadsheet.vi"("file path (dialog if empty)"=w368, "2D data"=w382) -> ("error out"=w367:errorcluster)  [unwired: 12 in, 1 out]
              n318 = call <vilib>:"Simple Error Handler.vi"("error in (no error)"=w367) -> ()  [unwired: 4 in, 5 out]
            }
          }
          n319 = case shown="真" w266 {
            tunnel: w265 -> [_ w345]
            frame False {
            }
            frame True {
              n320 = Index Array(array=w345, index=1 ("索引")) -> (element=w343:string)
              n321 = Decimal String To Number(string=w343) -> (number=w338:i32)  [unwired: 2 in, 1 out]
              n322 = Greater?(x=w338, y=10) -> (0:w340:bool)
              n323 = case shown="真" w340 {
                tunnel: [_ w356] -> w339
                tunnel: w338 -> [_ w357]
                frame False {
                  n324 = One Button Dialog(message="请输入大于6的数值" ("消息")) -> ()  [unwired: 1 in, 1 out]
                }
                frame True {
                  n325 = Subtract(x=w357, y=6) -> (x-y=w356:i32)
                }
              }
              n326 = Multiply(x=w339, y=1000) -> (x*y=→"x*y":i32)
              n327 = while {
                stop <- w346 stop-if-true
                n328 = local read "停止"() -> (w346:bool)
                n329 = case shown="假" w346 {
                  tunnel: [w350 11.0] -> w347
                  frame False {
                    n330 = Multiply(x="数据存储时间间隔（分钟）", y=60000.0) -> (x*y=w350:dbl)
                  }
                  frame True {
                  }
                }
                n331 = Wait (ms)(milliseconds to wait=w347) -> ()  [unwired: 1 out]
                n332 = flat-sequence {
                  frame #0 {
                    # "数据存储"
                    n333 = control-ref of="数据数组"() -> (w348:refnum<vi>)
                    n334 = call "数据存储(子VI).vi"("Array输入"=w348) -> ()  [unwired: 10 in, 1 out]
                  }
                  frame #1 {
                    # "数组初始化"
                    n335 = control-ref of="数据数组"() -> (w349:refnum<vi>)
                    n336 = call "数据初始化(子VI).vi"("Array输入"=w349) -> ()  [unwired: 10 in, 1 out]
                  }
                }
              }
            }
          }
          n337 = case shown="真" w304 {
            tunnel: w265 -> [_ w426]
            frame False {
            }
            frame True {
              n338 = Index Array(array=w426, index=1 ("索引")) -> (element=w428:string)
              n339 = Equal?(x=w428, y="1") -> (x = y?=w425:bool)
              n340 = case shown="真" w425 {
                frame False {
                  w430 = "" ("T(cool)℃")
                  n341 = local write "P（eq)mv"(w430) -> ()
                  n342 = local write "R(Gas)mv"(w430) -> ()
                  n343 = local write "T(cool)℃"(w430) -> ()
                }
                frame True {
                  # "读取流量传感器"
                  n344 = call "读取流量传感器(子VI).vi"() -> ("R(Gas)mv"=→"R(Gas)mv":string, "F(Flow)ml/min"=→"F(Flow)ml/min":string, "P（eq)mv"=→"P（eq)mv":string, "T(cool)℃"=→"T(cool)℃":string)  [unwired: 7 in, 1 out]
                }
              }
            }
          }
          n345 = Unbundle By Name(w298) -> ("status"=w280:bool)
          n346 = Unbundle By Name(w291) -> ("status"=w281:bool)
          n347 = Unbundle By Name(w292) -> ("status"=w282:bool)
          n348 = Unbundle By Name(w293) -> ("status"=w283:bool)
          n349 = Unbundle By Name(w294) -> ("status"=w286:bool)
          n350 = Unbundle By Name(w295) -> ("status"=w285:bool)
          n351 = case shown="真" w303 {
            tunnel: w265 -> [_ w406]
            tunnel: [_ w398] -> w290
            tunnel: [_ w397] -> w289
            tunnel: [_ w396] -> w288
            tunnel: [_ w395] -> w276
            frame False {
            }
            frame True {
              n352 = Index Array(array=w406, index=1 ("索引")) -> (element=w394:string)
              n353 = Equal?(x=w394, y="1") -> (x = y?=w405:bool)
              n354 = Equal?(x=w394, y="3") -> (x = y?=w404:bool)
              n355 = Equal?(x=w394, y="5") -> (x = y?=w402:bool)
              n356 = Equal?(x=w394, y="7") -> (x = y?=w400:bool)
              n357 = case shown="真" w405 {
                tunnel: [_ w422] -> w395
                tunnel: w394 -> [_ w421]
                frame False {
                }
                frame True {
                  n358 = local write "多位阀的位置"(w421) -> ()
                  n359 = call "VICI仪器串口通讯.vi"("输入指令"="CW1\n\r", "VISA resource name"=refnum<visa-resource-name> "COM1") -> ("错误输出"=w422:errorcluster)  [unwired: 1 in, 2 out]
                }
              }
              n360 = case shown="真" w404 {
                tunnel: [_ w418] -> w396
                tunnel: w394 -> [_ w417]
                frame False {
                }
                frame True {
                  n361 = local write "多位阀的位置"(w417) -> ()
                  n362 = call "VICI仪器串口通讯.vi"("输入指令"="CW3\n\r", "VISA resource name"=refnum<visa-resource-name> "COM1") -> ("错误输出"=w418:errorcluster)  [unwired: 1 in, 2 out]
                }
              }
              n363 = case shown="真" w402 {
                tunnel: [_ w414] -> w397
                tunnel: w394 -> [_ w413]
                frame False {
                }
                frame True {
                  n364 = local write "多位阀的位置"(w413) -> ()
                  n365 = call "VICI仪器串口通讯.vi"("输入指令"="CW5\n\r", "VISA resource name"=refnum<visa-resource-name> "COM1") -> ("错误输出"=w414:errorcluster)  [unwired: 1 in, 2 out]
                }
              }
              n366 = case shown="真" w400 {
                tunnel: [_ w410] -> w398
                tunnel: w394 -> [_ w409]
                frame False {
                }
                frame True {
                  n367 = local write "多位阀的位置"(w409) -> ()
                  n368 = call "VICI仪器串口通讯.vi"("输入指令"="CW7\n\r", "VISA resource name"=refnum<visa-resource-name> "COM1") -> ("错误输出"=w410:errorcluster)  [unwired: 1 in, 2 out]
                }
              }
            }
          }
          n369 = local read "停止"() -> (w256:bool)
          n370 = Unbundle By Name(w276) -> ("status"=w275:bool)
          n371 = Unbundle By Name(w288) -> ("status"=w277:bool)
          n372 = Unbundle By Name(w289) -> ("status"=w278:bool)
          n373 = Unbundle By Name(w290) -> ("status"=w279:bool)
          n374 = Build Array(w275, w277, w278, w279, w280, w281, w282, w283, w286, w285, w259) -> (w284:bool[])
          n375 = Or Array Elements(Boolean array=w284) -> (logical OR=w257:bool)
          n376 = Or(x=w256, y=w257) -> (x .or. y?=w255:bool)
        }
        n377 = Release Queue(queue=w194, error in (no error)=w185) -> ()  [unwired: 1 in, 3 out]
        "当前步骤" <- 0 ("数值")
        "跳转次数变量" <- 0 ("跳转次数变量")
      }
    }
    n378 = local write "停止"(w6) -> ()
    n379 = local write "停止"(w6) -> ()
    n380 = Unbundle By Name(T1 {"Row"=0, "Column"=5} ("活动单元格:活动单元格")) -> ("Row"=w17:i32, "Column"=w18:i32)
    n381 = Unbundle By Name(T1 {"Row"=0, "Column"=6} ("活动单元格:活动单元格")) -> ("Row"=w16:i32, "Column"=w15:i32)
    n382 = Unbundle By Name(T1 {"Row"=0, "Column"=3} ("活动单元格:活动单元格")) -> ("Row"=w25:i32, "Column"=w26:i32)
    n383 = Unbundle By Name(T1 {"Row"=0, "Column"=0} ("活动单元格:活动单元格")) -> ("Row"=w38:i32, "Column"=w37:i32)
    n384 = Unbundle By Name(T1 {"Row"=0, "Column"=2} ("活动单元格:活动单元格")) -> ("Row"=w30:i32, "Column"=w29:i32)
    n385 = Unbundle By Name(T1 {"Row"=0, "Column"=4} ("活动单元格:活动单元格")) -> ("Row"=w22:i32, "Column"=w21:i32)
    n386 = Unbundle By Name(T1 {"Row"=0, "Column"=7} ("活动单元格:活动单元格")) -> ("Row"=w11:i32, "Column"=w12:i32)
    n387 = Unbundle By Name(T1 {"Row"=0, "Column"=1} ("活动单元格:活动单元格")) -> ("Row"=w33:i32, "Column"=w34:i32)
    n388 = invoke on="步骤" class="Tbl (严格)" method="Set Cell Value (Deprecated)"("X Index"=w18, "Y Index"=w17, "Value"="参数2名称" ("值")) -> ()  [unwired: 3 in, 6 out]
    n389 = invoke on="步骤" class="Tbl (严格)" method="Set Cell Value (Deprecated)"("X Index"=w26, "Y Index"=w25, "Value"="参数1名称" ("值")) -> ()  [unwired: 3 in, 6 out]
    n390 = invoke on="步骤" class="Tbl (严格)" method="Set Cell Value (Deprecated)"("X Index"=w15, "Y Index"=w16, "Value"="参数2值" ("值")) -> ()  [unwired: 3 in, 6 out]
    n391 = invoke on="步骤" class="Tbl (严格)" method="Set Cell Value (Deprecated)"("X Index"=w37, "Y Index"=w38, "Value"="No" ("值")) -> ()  [unwired: 3 in, 6 out]
    n392 = invoke on="步骤" class="Tbl (严格)" method="Set Cell Value (Deprecated)"("X Index"=w29, "Y Index"=w30, "Value"="组合框" ("值")) -> ()  [unwired: 3 in, 6 out]
    n393 = invoke on="步骤" class="Tbl (严格)" method="Set Cell Value (Deprecated)"("X Index"=w21, "Y Index"=w22, "Value"="参数1值" ("值")) -> ()  [unwired: 3 in, 6 out]
    n394 = invoke on="步骤" class="Tbl (严格)" method="Set Cell Value (Deprecated)"("X Index"=w12, "Y Index"=w11, "Value"="Tip" ("值")) -> ()  [unwired: 3 in, 6 out]
    n395 = invoke on="步骤" class="Tbl (严格)" method="Set Cell Value (Deprecated)"("X Index"=w34, "Y Index"=w33, "Value"="设备" ("值")) -> ()  [unwired: 3 in, 6 out]
  }
  n396 = invoke on="步骤" class="Tbl (严格)" method="Reinit To Default"() -> ()  [unwired: 3 in, 3 out]
  n397 = local write "x*y"(6000 ("x*y")) -> ()
  n398 = control-ref of="数据数组"() -> (w1:refnum<vi>)
  n399 = call "数据初始化(子VI).vi"("Array输入"=w1) -> ()  [unwired: 10 in, 1 out]
  "输出数组 2" <- string[][] [["No", "设备", "组合框", "参数1名称", "参数1值", "参数2名称", "参数2值", "Tip"]] ("输出数组 2")
  "活动单元格:活动单元格" <- T1 {"Row"=0, "Column"=0} ("活动单元格:活动单元格")
  "数值 2" <- 0
